vi "Client Vision.vi"(11 "Channel Number":i32) -> (0 "error out":errorcluster)   [LabVIEW 2026]
uses:
  labview/auto-vision/Automotive Vision UI/Automotive-Vision-OOBService_client/RPC Messages/hwval_ExportRequest.ctl
  labview/auto-vision/Automotive Vision UI/Automotive-Vision-OOBService_client/Automotive-Vision-OOBService_client.lvlib
panel:
  in  "stop":bool
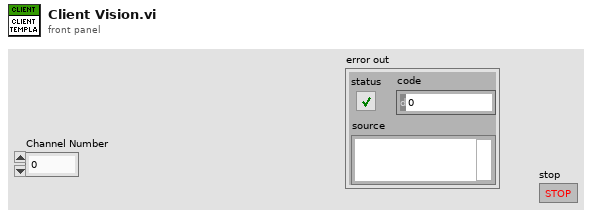
[diagram p1: front panel]
types:
  T1 = typedef "grpc-lvsupport-release.lvlib/grpcId.ctl" = u64
  T2 = typedef "Automotive-Vision-OOBService_client.lvlib/hwval_ExportRequest.ctl" = cluster{"FilePath":string}
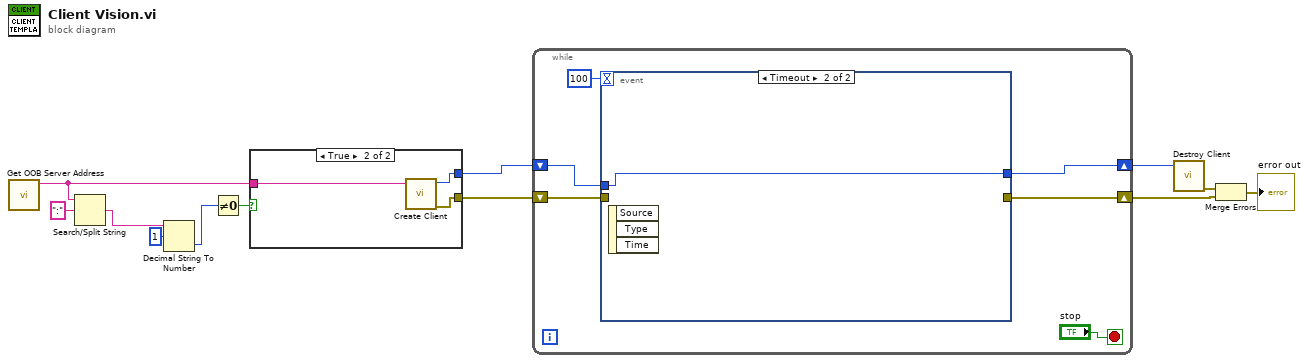
[diagram p0: block diagram]
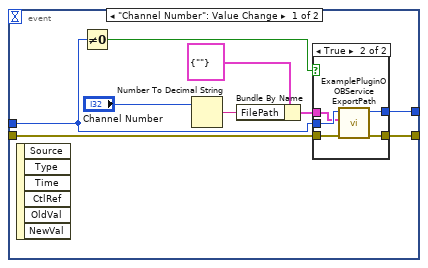
[diagram p2: hidden frame]
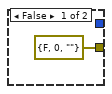
[diagram p4: hidden frame]
diagram:
  n1 = call "Get OOB Server Address.vi"() -> ("Address"=w5:string)  [unwired: 10 in, 1 out]
  n2 = Search/Split String(string=w5, search string/char (-)=":") -> (match + rest of string=w1:string)  [unwired: 1 in, 2 out]
  n3 = Decimal String To Number(string=w1, offset=1) -> (number=w3:i32)  [unwired: 1 in, 1 out]
  n4 = Not Equal To 0?(x=w3) -> (x != 0?=w12:bool)
  n5 = case shown="True" w12 {
    tunnel: [errorcluster {"status"=FALSE, "code"=0, "source"=""} ("error out") w15] -> w11
    tunnel: [_ w16] -> w10
    tunnel: w5 -> [_ w14]
    frame False {
    }
    frame True {
      n6 = call "Create Client.vi"("address"=w14) -> ("error out"=w15:errorcluster, "gRPC ID Out"=w16:T1)  [unwired: 9 in]
    }
  }
  n7 = while {
    shift-right: [w19] -> w6
    shift-left: w11 -> [w22]
    shift-right: [w20] -> w9
    shift-left: w10 -> [w21]
    stop <- "stop" stop-if-true
    n8 = event shown="[1] Timeout" {
      selector: _ -> [_ _]
      dyn-events: _ -> [_ _]
      timeout: 100 -> [_ _]
      tunnel: w22 -> [w26 _]
      tunnel: w21 -> [w25 w39]
      tunnel: [w24 w39] -> w20
      tunnel: [w23 _] -> w19
      event "Channel Number": Value Change {
        n9 = event-data() -> ()  [unwired: 1 in, 6 out]
        n10 = Not Equal To 0?(x=w25) -> (x != 0?=w30:bool)
        n11 = Number To Decimal String(number="Channel Number") -> (decimal integer string=w27:string)  [unwired: 1 in]
        n12 = Bundle By Name(cluster=T2 {"FilePath"=""} ("Request Data"), "FilePath"=w27) -> (w31:T2)
        n13 = case shown="True" w30 {
          tunnel: [w33 w35] -> w24
          tunnel: [w32 w37] -> w23
          tunnel: w25 -> [w33 w36]
          tunnel: w26 -> [w32 w38]
          tunnel: w31 -> [_ w34]
          frame False {
          }
          frame True {
            n14 = call "ExamplePluginOOBService ExportPath.vi"("error in"=w38, "Request Data"=w34, "gRPC ID"=w36) -> ("error out"=w37:errorcluster, "gRPC ID out"=w35:T1)  [unwired: 6 in, 1 out]
          }
        }
      }
      event Timeout {
        n15 = event-data() -> ()  [unwired: 1 in, 3 out]
      }
    }
  }
  n16 = call "Destroy Client.vi"("gRPC ID"=w9) -> ("error out"=w8:errorcluster)  [unwired: 10 in]
  n17 = Merge Errors(w8, w6) -> (→"error out":errorcluster)
